vi "Initialize UDP.vi"(8 "error in":errorcluster, 11 "UDP In":refnum<class "UDP.lvclass">) -> (0 "error out":errorcluster, 3 "UDP out":refnum<class "UDP.lvclass">)   [LabVIEW 2018, in "UDP.lvlib" / "UDP.lvclass"]
uses:
  UDP.lvclass
  C:/AME Test Engineering/LabVIEW/PPLs/LiDAR/Parent/LiDAR.lvlibp/LiDAR.lvclass
  UDP.lvclass/UDP.ctl
  PPLs/Configuration/Configuration.lvlibp/Configuration.lvclass
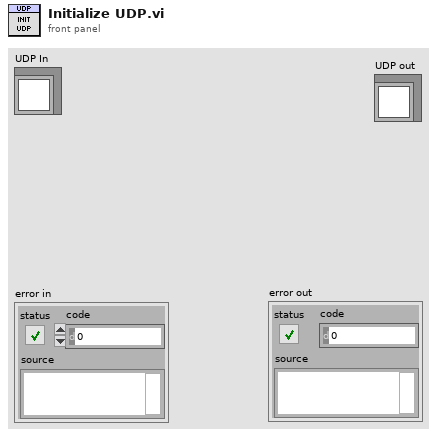
[diagram p1: front panel]
types:
  T1 = cluster{"Configuration":refnum<class "Configuration.lvclass">, "Network":cluster{"TCP":cluster{"IP Address":string, "Port":u16}, "UDP":cluster{"IP Address":string, "Port":u16}}, "Azimuth":cluster{"Min >=-60":string, "Max <=+60":string}, "Elevation":cluster{"FOV":string, "Offset":string, "Scan Pattern":enum16{"Triangle", "Snap"}, "Frequency":string}, "Data Algo":enum16{"Resim", "Point Cloud"}}
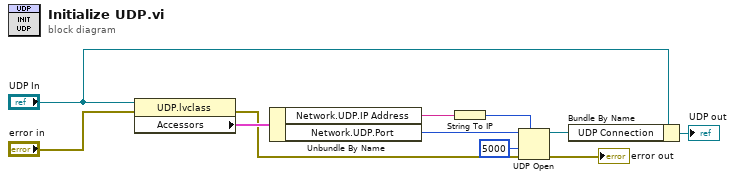
[diagram p0: block diagram]
diagram:
  n1 = property class="UDP.lvclass"(reference="UDP In", error in="error in") -> (error out=w5:errorcluster, "Accessors"=w11:T1)  [unwired: 1 out]
  n2 = Unbundle By Name(w11) -> ("Network.UDP.IP Address"=w9:string, "Network.UDP.Port"=w10:u16)
  n3 = String To IP(1:w9) -> (0:w8:u32)
  n4 = UDP Open(7:w8, 8:w5, 9:5000 ("timeout ms (25000)"), 11:w10) -> (port=w2:refnum<k16>, 0:→"error out":errorcluster)  [unwired: 1 in, 1 out]
  n5 = Bundle By Name(cluster="UDP In", "UDP Connection"=w2) -> (→"UDP out":refnum<class "UDP.lvclass">)
